vi "test.vi"() -> ()   [LabVIEW 2019]
uses:
  <vilib>/Platform/TimedLoop/XDataNode/timing_clust.ctl
  <vilib>/Platform/TimedLoop/XDataNode/nitl_modes.ctl
  <vilib>/Platform/TimedLoop/XDataNode/wakeup.ctl
  <extravilib>/ChannelInstances/Tag-bool/Read With Abort.vi
  <extravilib>/ChannelInstances/Tag-bool/Write With Abort.vi
  <vilib>/Plasmionique/MB Master/MB_Master_TCP/MB_Master_TCP.lvclass
  C:/Program Files (x86)/National Instruments/LabVIEW 2019/vi.lib/Plasmionique/MB Master/MB_Master/MB_Master.lvclass
  <extravilib>/ChannelInstances/Tag-bool/Instantiate.vi
  <extravilib>/ChannelInstances/Tag-bool/EndpointRead.vi
  <extravilib>/ChannelInstances/Tag-bool/Endpoint.vi
  <vilib>/Platform/TimedLoop/XDataNode/XDataNode.xnode
  <vilib>/Platform/TimedLoop/XDataNode/XDNodeRunTimeDep.lvlib
  <extravilib>/ChannelInstances/Tag-bool.lvlib
  <vilib>/Plasmionique/MB Master/MB Master.lvlib
  <instrlib>/Sefram DAS240/Sefram DAS240.lvlib
panel:
  in  "VISA resource name":refnum<visa-resource-name>
  out "error out":errorcluster
  in  "Chemin de sortie":path=path "C:/Users/manip/Documents/Thermo aquisition data/labview/output"
  in  "Nom de l'analyse":string="sys1_isoPlac_"
  in  "Fréequence \nd'échantillonage (alim)":dbl=1.0 caption="Fréequence d'échantillonage (Hz)"
  in  "Generation de données":enum32{"Labview", "CSV"}(tab)
  in  "Labview opt":T1={"Fréequence maximale (Hz)"=0.1, "Temps de simulation (min)"=2.0, "Amplitude minimale (V)"=0.0, "Amplitude maximale (V)"=1.0}
  in  "Chemin du fichier":path=path "C:/Users/manip/Documents/Thermo aquisition data/labview/input/data.csv"
  out "DSP par FFT":cluster{dbl[], dbl[]}(graph)
  out "Signal d'entrée":cluster{dbl[], dbl[]}(graph)
  in  "START":bool
  in  "Generer nouveau":bool
  out "Haute temperature":bool
  in  "Température maximale":dbl=100.0 caption="Fréequence d'échantillonage (Hz)"
  out "Prêt":bool
  out "Signal d'entrée mesuré":sgl(graph)
  out "Signal de sortie":sgl(graph)
  in  "stop":bool
  out "Das trouvé":bool
  out "Alim connectée":bool
  in  "Numéro de la machine voulu":string="2196400002"
  out "Machines trouvées":string[][](array[string])=[["COM7", "PSI 9200-25", "2196400002", "06230310", "", "200,0000", "25,0000", "1500,0000", "0,0000", "240,0000", "33", "PSI 9000 Series", "0", "", "", "", "", "V2.31 24.08.2020", "V2.20 20.11.2020", "V1.6.6", "Modbus_RTU"], ["TCPIP0::169.254.133.212::502::SOCKET", "", "", "", "///", "0,000", "0,000", "0,000", "", "", "0", "Ethernet", "0", "", "", "", "", "", "", "", "Can"]]
  out "Sortie d'erreur":errorcluster
  in  "Adresse IP":string="169.254.133.212"
  in  "Fréequence d'échantillonage \n(aquisition)":dbl=10.0 caption="Fréequence d'échantillonage (Hz)"
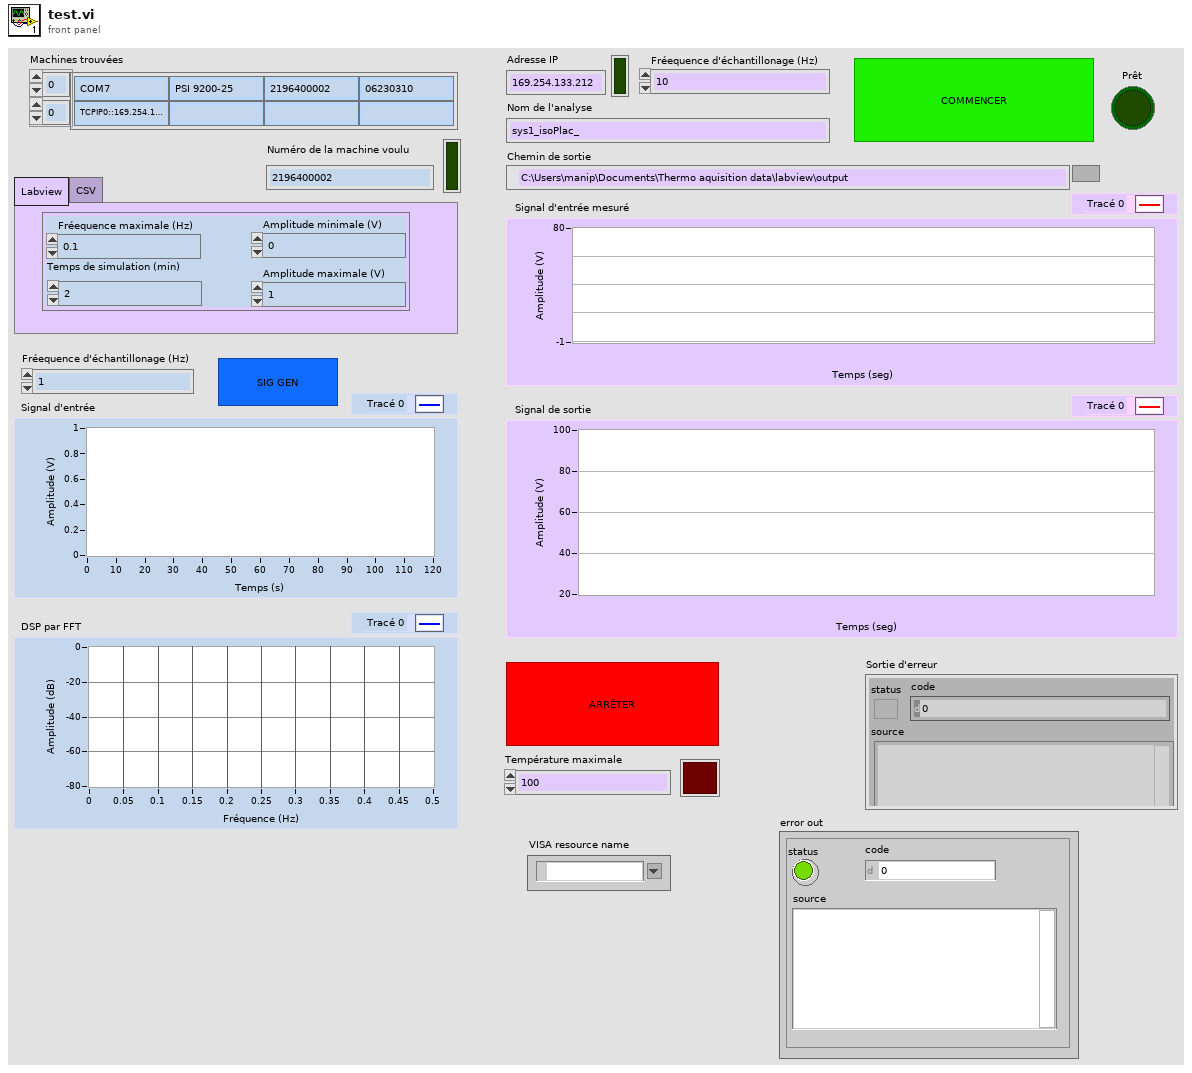
[diagram p1: front panel]
types:
  T1 = cluster{"Fréequence maximale (Hz)":dbl, "Temps de simulation (min)":dbl, "Amplitude minimale (V)":dbl, "Amplitude maximale (V)":dbl}
  T2 = typedef "XDNodeRunTimeDep.lvlib/timing_clust.ctl" = cluster{"Expected End [f-1]":u64, "Actual End [f-1]":u64, "Finished Late? [f-1]":bool, "Expected End [i-1]":u64, "Actual End [i-1]":u64, "Finished Late? [i-1]":bool, "Expected Start [i]":u64, "Actual Start [i]":u64, "Expected Start [f]":u64, "Actual Start [f]":u64, "Source Name":string, "Structure Name":string, "Period":i64, "Deadline":i64, "Offset":i64, "Start":i64, "Priority":i32, "Timeout":i32, "Mode":T3, "Wakeup Reason":T4, "Error":errorcluster, "Source Type":string, "Secondary Source Type":string, "Global End Time":u64, "Global Start Time":u64, "Frame Duration":u64, "Iteration Duration":u64, "Assigned CPU":i32, "I/O Scan Engine Mode":u32}
  T3 = typedef "XDNodeRunTimeDep.lvlib/nitl_modes.ctl" = enum32{"No Change", "Process missed periods, maintain original phase", "Discard missed periods, maintain original phase", "Process missed periods, ignore original phase", "Discard missed periods, ignore original phase"}
  T4 = typedef "XDNodeRunTimeDep.lvlib/wakeup.ctl" = enum32{"Normal", "Aborted", "Asynchronous wakeup", "Timing source error", "Timed loop error", "Timeout"}
  T5 = typedef "Tag-bool.lvlib/))Channel.ctl" = refnum<queue>
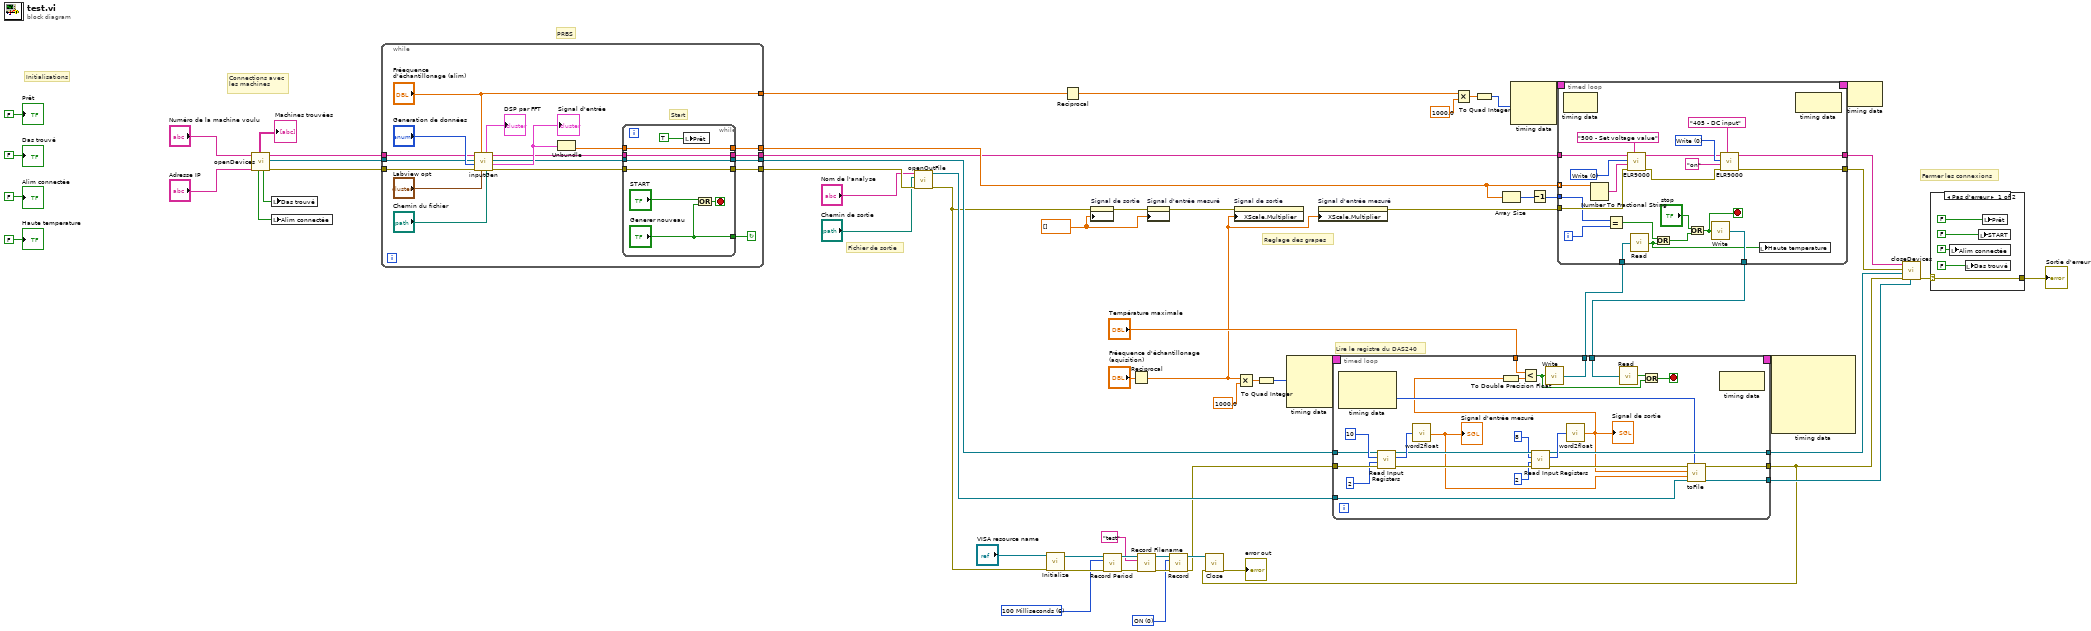
[diagram p0: block diagram]
diagram:
  w4 = u16 0 items=["ON", "OFF", "TRIG"] ("Record State")
  w11 = u16 6 items=["1 Millisecond", "2 Milliseconds", "5 Milliseconds", "10 Milliseconds", "20 Milliseconds", "50 Milliseconds", "100 Milliseconds", "200 Milliseconds", "500 Milliseconds", "1 Second", "2 Seconds", "5 Seconds", "10 Seconds", "20 Seconds", "1 Minute", "2 Minutes", "5 Minutes", "10 Minutes", "20 Minutes"] ("Record Period")
  w35 = sgl[] [] ("Données d'historique")
  # "PRBS"
  # "Fichier de sortie"
  # "Initialisations"
  # "Reglage des grapes"
  # "Fermer les connexions"
  # "Lire le registre du DAS240"
  # "Connections avec\nles machines"
  n1 = call "openDevices.vi"("Adresse IP (DAS240)"="Adresse IP", "Numéro de série (PSI - 9200)"="Numéro de la machine voulu") -> ("Erreur de sortie"=w24:errorcluster, "DAS240_ID"=w23:refnum<class "MB_Master_TCP.lvclass">, "PSI_ID"=w22:string[], "Das trouvé"=w31:bool, "Alim connectée"=w30:bool, "Machines trouvées"=→"Machines trouvées":string[][])  [unwired: 4 in]
  n2 = local write "Das trouvé"(w31) -> ()
  n3 = local write "Alim connectée"(w30) -> ()
  n4 = while {
    tunnel: ["Fréequence \nd'échantillonage (alim)"] -> w46
    tunnel: [w72] -> w41
    tunnel: w24 -> [w71]
    tunnel: w23 -> [w70]
    tunnel: w22 -> [w69]
    tunnel: [w68] -> w19
    tunnel: [w67] -> w21
    tunnel: [w66] -> w20
    stop <- w64 continue-if-true
    # "Start"
    n5 = call "inputGen.vi"("Chemin du fichier"="Chemin du fichier", "Labview opt"="Labview opt", "Fréequence \nd'échantillonage (alim)"="Fréequence \nd'échantillonage (alim)", "Entrée d'erreur"=w71, "Commande onglets"="Generation de données", "DAS240_ID IN"=w70, "PSI_ID IN"=w69) -> ("Sortie d'erreur"=w65:errorcluster, "Signal d'entrée"=w76:cluster{dbl[], dbl[]}, "DAS240_ID OUT"=w74:refnum<class "MB_Master_TCP.lvclass">, "PSI_ID OUT"=w75:string[], "DSP par FFT"=→"DSP par FFT":cluster{dbl[], dbl[]})
    "Signal d'entrée" <- w76
    n6 = Unbundle(w76) -> (w73:dbl[])  [unwired: 1 out]
    n7 = while {
      tunnel: w75 -> [w89]
      tunnel: [w89] -> w67
      tunnel: [w88] -> w66
      tunnel: w74 -> [w88]
      tunnel: [w87] -> w72
      tunnel: w73 -> [w87]
      tunnel: [w86] -> w68
      tunnel: w65 -> [w86]
      tunnel: ["Generer nouveau"] -> w64
      stop <- w84 stop-if-true
      n8 = local write "Prêt"(TRUE ("START")) -> ()
      n9 = Or(x="START", y="Generer nouveau") -> (x .or. y?=w84:bool)
    }
  }
  n10 = call "openOutFile.vi"("Entrée d'erreur"=w19, "Chemin de sortie"="Chemin de sortie", "Nom de l'analyse"="Nom de l'analyse") -> ("Sortie d'erreur"=w3:errorcluster, "refnum en sortie"=w16:refnum<file>)  [unwired: 6 in, 1 out]
  n11 = call <instrlib>:"Initialize.vi"("error in (no error)"=w3, "VISA resource name"="VISA resource name") -> ("error out"=w14:errorcluster, "VISA resource name out"=w15:refnum<visa-resource-name>)  [unwired: 8 in]
  n12 = Reciprocal(x=w46) -> (1/x=w34:dbl)
  n13 = property on="Signal de sortie" class="GraphDér (strict)"(error in=w3, "History Data"=w35) -> (error out=w27:errorcluster)  [unwired: 1 in, 1 out]
  n14 = call <instrlib>:"Record Period.vi"("error in (no error)"=w14, "Record Period"=w11, "VISA resource name"=w15) -> ("error out"=w9:errorcluster, "VISA resource name out"=w10:refnum<visa-resource-name>)  [unwired: 7 in]
  n15 = Reciprocal(x="Fréequence d'échantillonage \n(aquisition)") -> (1/x=w28:dbl)
  n16 = call <instrlib>:"Record Filename.vi"("error in (no error)"=w9, "Filename"="test", "VISA resource name"=w10) -> ("error out"=w6:errorcluster, "VISA resource name out"=w7:refnum<visa-resource-name>)  [unwired: 7 in]
  n17 = property on="Signal d'entrée mesuré" class="GraphDér (strict)"(error in=w27, "History Data"=w35) -> (error out=w25:errorcluster)  [unwired: 1 in, 1 out]
  n18 = call <instrlib>:"Record.vi"("error in (no error)"=w6, "Record State"=w4, "VISA resource name"=w7) -> ("error out"=w2:errorcluster, "VISA resource name out"=w5:refnum<visa-resource-name>)  [unwired: 7 in]
  n19 = property on="Signal de sortie" class="GraphDér (strict)"(error in=w25, "XScale.Multiplier"=w28) -> ()  [unwired: 1 in, 2 out]
  n20 = Multiply(x=w28, y=1000.0) -> (x*y=w55:dbl)
  n21 = To Quad Integer(1:w55) -> (0:w53:i64)
  n22 = node-c288(w53) -> (w61:T2)  [unwired: 3 in]
  n23 = property on="Signal d'entrée mesuré" class="GraphDér (strict)"("XScale.Multiplier"=w28) -> (error out=w26:errorcluster)  [unwired: 2 in, 1 out]
  n24 = Multiply(x=w34, y=1000.0) -> (x*y=w58:dbl)
  n25 = To Quad Integer(1:w58) -> (0:w57:i64)
  n26 = Array Size(array=w41) -> (size(s)=w40:i32)
  n27 = node-c288(w57) -> (w63:T2)  [unwired: 2 in]
  n28 = Decrement(x=w40) -> (x-1=w39:i32)
  n29 = call <instrlib>:"Close.vi"("error in (no error)"=w1, "VISA resource name"=w5) -> ("error out"=→"error out":errorcluster)  [unwired: 9 in]
  n30 = timed-loop {
    timing: w61 -> [_]
    timing-out: [_] -> w60
    tunnel: w20 -> [w106]
    tunnel: w2 -> [w114]
    tunnel: [w102] -> w1
    tunnel: [w108] -> w47
    tunnel: w45 -> [w103]
    tunnel: w16 -> [w100]
    tunnel: [w99] -> w42
    tunnel: [w96] -> w38
    tunnel: "Température maximale" -> [w92]
    stop <- w93 stop-if-true
    n31 = node-c288() -> (w97:i64)  [unwired: 1 in, 2 out]
    n32 = call <vilib>:"Read Input Registers.vi"("error in (no error)"=w114, "quantity"=u16 2, "starting address"=u16 10, "MB session in"=w106) -> ("error out"=w109:errorcluster, "Registers"=w110:u16[], "MB session out"=w107:refnum<class "MB_Master_TCP.lvclass">)  [unwired: 5 in]
    n33 = call "word2float.vi"("Tableau d'entrée"=w110) -> ("Float de sortie"=w98:sgl)
    "Signal d'entrée mesuré" <- w98
    n34 = call <vilib>:"Read Input Registers.vi"("error in (no error)"=w109, "quantity"=u16 2, "starting address"=u16 8, "MB session in"=w107) -> ("error out"=w101:errorcluster, "Registers"=w111:u16[], "MB session out"=w108:refnum<class "MB_Master_TCP.lvclass">)  [unwired: 5 in]
    n35 = call "word2float.vi"("Tableau d'entrée"=w111) -> ("Float de sortie"=w90:sgl)
    "Signal de sortie" <- w90
    n36 = To Double Precision Float(number=w90) -> (double precision float=w91:dbl)
    n37 = Less?(x=w92, y=w91) -> (x < y?=w94:bool)
    n38 = call <extravilib>:"Write.vi"("element"=w94) -> ("channel"=w96:T5)  [unwired: 1 out]
    n39 = call <extravilib>:"Read.vi"("channel"=w103) -> ("element"=w95:bool)  [unwired: 1 in, 1 out]
    n40 = Or(x=w95, y=w94) -> (x .or. y?=w93:bool)
    n41 = call "toFile.vi"("Temps t"=w97, "refnum"=w100, "Tension u"=w98, "Temp y"=w90, "entrée d'erreur"=w101) -> ("refnum en sortie"=w99:refnum<file>, "sortie d'erreur"=w102:errorcluster)  [unwired: 5 in]
    n42 = node-c288() -> ()  [unwired: 1 in, 1 out]
  }
  n43 = timed-loop {
    timing: w63 -> [_]
    timing-out: [_] -> w62
    tunnel: w21 -> [w129]
    tunnel: w26 -> [w131]
    tunnel: [w119] -> w48
    tunnel: [w130] -> w49
    tunnel: w41 -> [w128] mode=indexing
    tunnel: [w127] -> w45
    tunnel: w39 -> [w126]
    tunnel: w38 -> [w120]
    i -> [w125]
    stop <- w124 stop-if-true
    w137 = u8 0 items=["Write", "Read"] ("Access")
    w139 = u8 0 items=["Write", "Read"] ("Access")
    n44 = node-c288() -> ()  [unwired: 1 in, 1 out]
    n45 = Number To Fractional String(number=w128) -> (F-format string=w132:string)  [unwired: 3 in]
    n46 = Equal?(x=w126, y=w125) -> (x = y?=w121:bool)
    n47 = call <instrlib>:"ELR9000.vi"("Command list"="500 - Set voltage value", "Error in"=w131, "Value"=w132, "Access"=w139, "Device information in"=w129) -> ("Error out"=w134:errorcluster, "Device information out"=w135:string[])  [unwired: 1 in, 2 out]
    n48 = call <extravilib>:"Read.vi"("channel"=w120) -> ("element"=w118:bool)  [unwired: 1 in, 1 out]
    n49 = Or(x=w121, y=w118) -> (x .or. y?=w122:bool)
    n50 = Or(x="stop", y=w122) -> (x .or. y?=w124:bool)
    n51 = call <extravilib>:"Write.vi"("element"=w124) -> ("channel"=w127:T5)  [unwired: 1 out]
    n52 = call <instrlib>:"ELR9000.vi"("Command list"="405 - DC input", "Error in"=w134, "Value"="on", "Access"=w137, "Device information in"=w135) -> ("Error out"=w119:errorcluster, "Device information out"=w130:string[])  [unwired: 1 in, 2 out]
    n53 = local write "Haute temperature"(w118) -> ()
    n54 = node-c288() -> ()  [unwired: 1 in, 1 out]
  }
  n55 = node-c288(w60) -> ()  [unwired: 7 out]
  n56 = node-c288(w62) -> ()  [unwired: 1 out]
  n57 = call "closeDevices.vi"("Fichier"=w42, "Erreur d'entrée DAS"=w1, "MB TCP session"=w47, "Erreur d'entrée alim"=w48, "Device information in"=w49) -> ("Erreur de sortie"=w44:errorcluster)  [unwired: 6 in]
  n58 = case shown="Pas d'erreur" w44 {
    selector: w44 -> [w146 w147]
    tunnel: [w146 w147] -> w36
    frame No Error {
      n59 = local write "Alim connectée"(FALSE ("element")) -> ()
      n60 = local write "Das trouvé"(FALSE ("element")) -> ()
      n61 = local write "START"(FALSE ("element")) -> ()
      n62 = local write "Prêt"(FALSE ("element")) -> ()
    }
    frame Error {
    }
  }
  "Sortie d'erreur" <- w36
  "Alim connectée" <- FALSE ("Alim connectée")
  "Das trouvé" <- FALSE ("Das trouvé")
  "Prêt" <- FALSE ("Ready")
  "Haute temperature" <- FALSE ("Haute temperature")
